vi "ServoControl_myrio_v3.vi"() -> ()   [LabVIEW 2019]
uses:
  <vilib>/Platform/TimedLoop/XDataNode/timing_clust.ctl
  <vilib>/Platform/TimedLoop/XDataNode/nitl_modes.ctl
  <vilib>/Platform/TimedLoop/XDataNode/wakeup.ctl
  <vilib>/Instr/_visa.llb/VISA Configure Serial Port (Instr).vi
  <vilib>/platform/TimedLoop/XDataNode/XDataNode.xnode
  <vilib>/Platform/TimedLoop/XDataNode/XDNodeRunTimeDep.lvlib
panel:
  in  "stop":bool
  in  "Loop Period":i64=5
  in  "sinewave period":dbl=10.0
  out "Servo Position Graph":cluster{dbl[], dbl[]}[](graph)
  in  "graph plot freq.":i32=1
  in  "const(f)/sine(t)":bool
  out "iteration":i32
  out "time":dbl
  out "sine position":dbl
  out "read from visa":string
  out "write to visa":string
  in  "const posotion":dbl=180.0
  in  "VISA resource name":refnum<visa-resource-name>="ASRL2::INSTR"
  in  "baud rate (9600)":u32=500000
  out "error out":errorcluster
  # "Servo motor"
  # "Read data to csv file"
  # "visa setting"
  # "servo setting"
  # "Timed loop status"
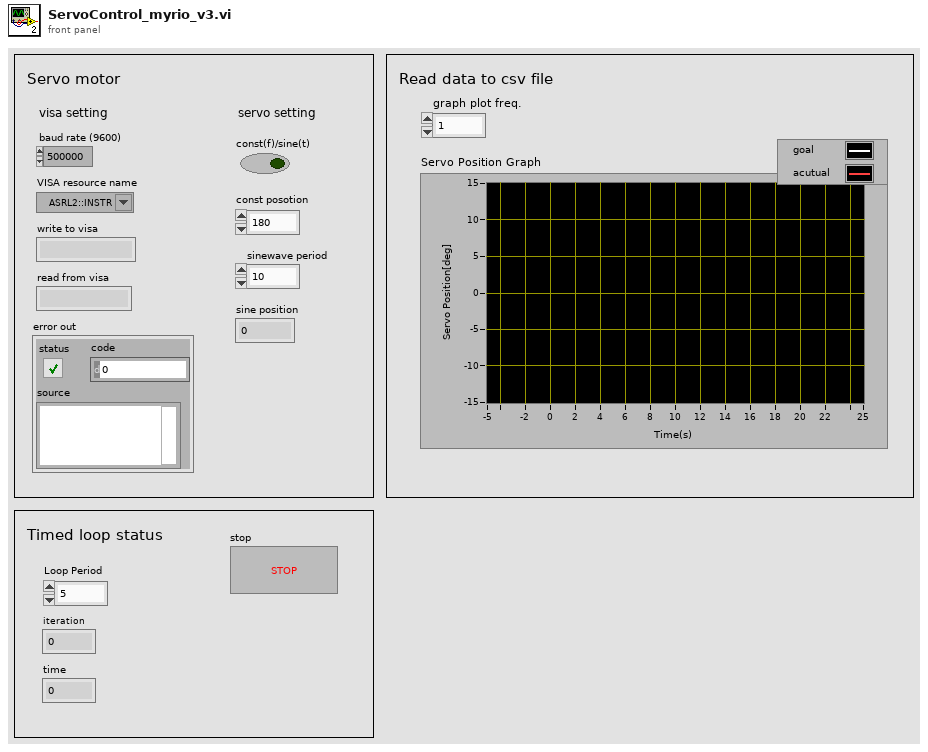
[diagram p1: front panel]
types:
  T1 = typedef "XDNodeRunTimeDep.lvlib/timing_clust.ctl" = cluster{"Expected End [f-1]":u64, "Actual End [f-1]":u64, "Finished Late? [f-1]":bool, "Expected End [i-1]":u64, "Actual End [i-1]":u64, "Finished Late? [i-1]":bool, "Expected Start [i]":u64, "Actual Start [i]":u64, "Expected Start [f]":u64, "Actual Start [f]":u64, "Source Name":string, "Structure Name":string, "Period":i64, "Deadline":i64, "Offset":i64, "Start":i64, "Priority":i32, "Timeout":i32, "Mode":T2, "Wakeup Reason":T3, "Error":errorcluster, "Source Type":string, "Secondary Source Type":string, "Global End Time":u64, "Global Start Time":u64, "Frame Duration":u64, "Iteration Duration":u64, "Assigned CPU":i32, "I/O Scan Engine Mode":u32}
  T2 = typedef "XDNodeRunTimeDep.lvlib/nitl_modes.ctl" = enum32{"No Change", "Process missed periods, maintain original phase", "Discard missed periods, maintain original phase", "Process missed periods, ignore original phase", "Discard missed periods, ignore original phase"}
  T3 = typedef "XDNodeRunTimeDep.lvlib/wakeup.ctl" = enum32{"Normal", "Aborted", "Asynchronous wakeup", "Timing source error", "Timed loop error", "Timeout"}
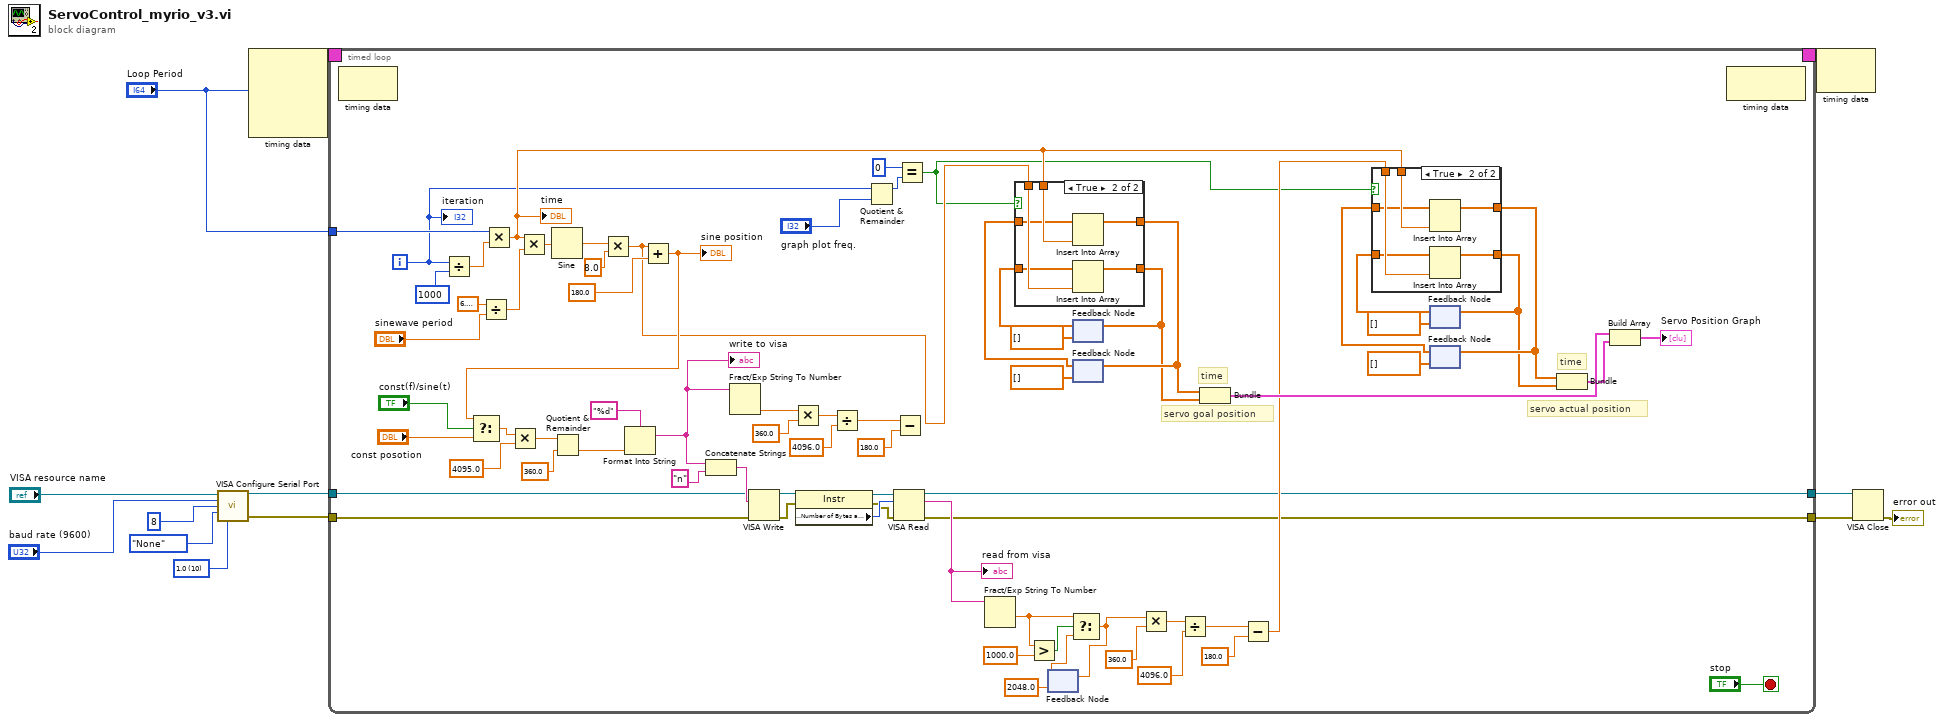
[diagram p0: block diagram]
diagram:
  w10 = u16 10 items=["1.0"=10, "1.5"=15, "2.0"=20] ("stop bits (10: 1 bit)")
  n1 = call-poly "VISA Configure Serial Port"("VISA resource name"="VISA resource name", "baud rate (9600)"="baud rate (9600)", "data bits (8)"=u16 8, "parity (0:none)"=enum16{"None", "Odd", "Even", "Mark", "Space"}."None", "stop bits (10: 1 bit)"=w10) -> ("VISA resource name out"=w3:refnum<visa-resource-name>, "error out"=w2:errorcluster)  [unwired: 9 in]
  n2 = node-c288("Loop Period") -> (w7:T1)  [unwired: 3 in]
  n3 = timed-loop {
    timing: w7 -> [_]
    timing-out: [_] -> w6
    tunnel: [w20] -> w5
    tunnel: [w19] -> w4
    tunnel: w3 -> [w18]
    tunnel: w2 -> [w17]
    tunnel: "Loop Period" -> [w16]
    i -> [w15]
    stop <- "stop" stop-if-true
    # "time"
    # "servo actual position"
    # "time"
    # "servo goal position"
    n4 = node-c288() -> ()  [unwired: 1 in, 1 out]
    n5 = Divide(x=w15, y=i64 1000) -> (x/y=w65:dbl)
    n6 = Divide(x=6.283185307179586, y="sinewave period") -> (x/y=w26:dbl)
    n7 = Multiply(x=w16, y=w65) -> (x*y=w22:dbl)
    "time" <- w22
    n8 = Multiply(x=w22, y=w26) -> (x*y=w68:dbl)
    n9 = Sine(x=w68) -> (sin(x)=w53:dbl)
    n10 = Multiply(x=w53, y=8.0) -> (x*y=w23:dbl)
    n11 = Add(x=w23, y=180.0) -> (x+y=w63:dbl)
    "sine position" <- w63
    n12 = Select(t=w63, s="const(f)/sine(t)", f="const posotion") -> (s? t:f=w61:dbl)
    n13 = Multiply(x=w61, y=4095.0) -> (x*y=w84:dbl)
    n14 = Quotient & Remainder(x=w84, y=360.0) -> (floor(x/y)=w82:dbl)  [unwired: 1 out]
    n15 = Format Into String(format string="%d", w82) -> (resulting string=w75:string)  [unwired: 2 in, 1 out]
    "write to visa" <- w75
    n16 = Concatenate Strings(w75, "n" ("string")) -> (w86:string)
    n17 = Fract/Exp String To Number(string=w75) -> (number=w74:dbl)  [unwired: 3 in, 1 out]
    n18 = VISA Write(VISA resource name=w18, write buffer=w86, error in (no error)=w17) -> (VISA resource name out=w51:refnum<visa-resource-name>, error out=w50:errorcluster)  [unwired: 1 out]
    n19 = Multiply(x=w74, y=360.0 ("x")) -> (x*y=w72:dbl)
    n20 = property class="Instr"(reference=w51, error in=w50) -> (reference out=w48:refnum<visa-resource-name>, error out=w47:errorcluster, "Serial Settings:Number of Bytes at Serial Port"=w49:u32)
    n21 = Divide(x=w72, y=4096.0) -> (x/y=w77:dbl)
    n22 = Quotient & Remainder(x=w15, y="graph plot freq.") -> (x-y*floor(x/y)=w56:i32)  [unwired: 1 out]
    n23 = VISA Read(VISA resource name=w48, byte count=w49, error in (no error)=w47) -> (VISA resource name out=w19:refnum<visa-resource-name>, read buffer=w76:string, error out=w20:errorcluster)  [unwired: 1 out]
    "read from visa" <- w76
    n24 = Subtract(x=w77, y=180.0) -> ()  [unwired: 1 out]
    n25 = Equal?(x=0, y=w56) -> (x = y?=w21:bool)
    n26 = Fract/Exp String To Number(string=w76) -> (number=w46:dbl)  [unwired: 3 in, 1 out]
    n27 = Greater?(x=w46, y=1000.0) -> (0:w45:bool)
    n28 = feedback #1(2048.0) -> (w30:dbl)
    n29 = Select(t=w46, s=w45, f=w30) -> (s? t:f=w31:dbl)
    n30 = feedback-in #1(w31) -> ()
    n31 = feedback #2(dbl[] []) -> (w60:dbl[])
    n32 = feedback #3(dbl[] []) -> (w57:dbl[])
    n33 = case shown="True" w21 {
      tunnel: w22 -> [_ w102]
      tunnel: w23 -> [_ w101]
      tunnel: [w96 w100] -> w24
      tunnel: w60 -> [w96 w99]
      tunnel: [w95 w98] -> w25
      tunnel: w57 -> [w95 w97]
      frame False {
      }
      frame True {
        n34 = Insert Into Array(array=w97, new element=w102) -> (w98:dbl[])  [unwired: 1 in]
        n35 = Insert Into Array(array=w99, new element=w101) -> (w100:dbl[])  [unwired: 1 in]
      }
    }
    n36 = feedback-in #2(w24) -> ()
    n37 = feedback-in #3(w25) -> ()
    n38 = Multiply(x=w31, y=360.0 ("x")) -> (x*y=w69:dbl)
    n39 = Divide(x=w69, y=4096.0) -> (x/y=w71:dbl)
    n40 = Bundle(w25, w24) -> (w40:cluster{dbl[], dbl[]})  [unwired: 1 in]
    n41 = Subtract(x=w71, y=180.0) -> (x-y=w35:dbl)
    n42 = feedback #4(dbl[] []) -> (w44:dbl[])
    n43 = feedback #5(dbl[] []) -> (w41:dbl[])
    n44 = case shown="True" w21 {
      tunnel: w22 -> [_ w94]
      tunnel: w35 -> [_ w93]
      tunnel: [w88 w92] -> w36
      tunnel: w44 -> [w88 w91]
      tunnel: [w87 w90] -> w37
      tunnel: w41 -> [w87 w89]
      frame False {
      }
      frame True {
        n45 = Insert Into Array(array=w89, new element=w94) -> (w90:dbl[])  [unwired: 1 in]
        n46 = Insert Into Array(array=w91, new element=w93) -> (w92:dbl[])  [unwired: 1 in]
      }
    }
    n47 = feedback-in #4(w36) -> ()
    n48 = feedback-in #5(w37) -> ()
    n49 = Bundle(w37, w36) -> (w39:cluster{dbl[], dbl[]})  [unwired: 1 in]
    n50 = Build Array(w40, w39) -> (→"Servo Position Graph":cluster{dbl[], dbl[]}[])
    n51 = node-c288() -> ()  [unwired: 1 in, 1 out]
    "iteration" <- w15
  }
  n52 = node-c288(w6) -> ()  [unwired: 1 out]
  n53 = VISA Close(VISA resource name=w4, error in (no error)=w5) -> (error out=→"error out":errorcluster)
